vi "Create Read Write Stream.vi"(8 "error in (no error)":errorcluster, 10 "IP":string, 11 "Channel in":refnum<class "Channel.lvclass">) -> (0 "error out":errorcluster, 3 "Channel out":refnum<class "Channel.lvclass">)   [LabVIEW 2018, in "Channel.lvclass"]
uses:
  Channel.lvclass
  Stream/Stream.lvclass
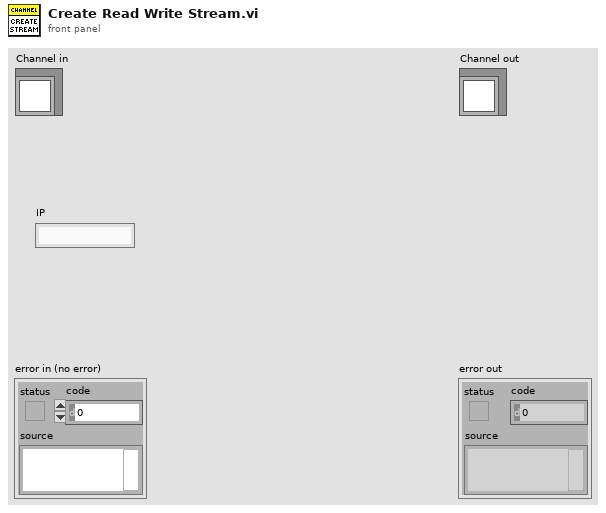
[diagram p1: front panel]
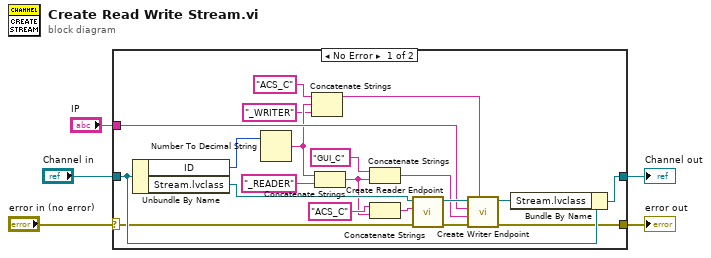
[diagram p0: block diagram]
diagram:
  n1 = case shown="No Error" "error in (no error)" {
    selector: "error in (no error)" -> [w23 w27]
    tunnel: [w20 w27] -> w4
    tunnel: [w24 w26] -> w2
    tunnel: "Channel in" -> [w25 w26]
    tunnel: "IP" -> [w17 _]
    frame No Error {
      n2 = Unbundle By Name(w25) -> ("ID"=w6:u8, "Stream.lvclass"=w22:refnum<class "Stream.lvclass">)
      n3 = Number To Decimal String(number=w6) -> (decimal integer string=w9:string)  [unwired: 1 in]
      n4 = Concatenate Strings("ACS_C" ("writer name"), w9, "_WRITER" ("writer name")) -> (w7:string)
      n5 = Concatenate Strings(w9, "_READER" ("writer name")) -> (w12:string)
      n6 = Concatenate Strings("GUI_C" ("writer name"), w12) -> (w11:string)
      n7 = Concatenate Strings("ACS_C" ("writer name"), w12) -> (w14:string)
      n8 = call "Create Reader Endpoint.vi"("error in (no error)"=w23, "reader name"=w14, "Stream in"=w22) -> ("error out"=w19:errorcluster, "Stream out"=w18:refnum<class "Stream.lvclass">)  [unwired: 7 in]
      n9 = call "Create Writer Endpoint.vi"(7:w7, "error in (no error)"=w19, "reader name"=w11, "IP"=w17, "Stream in"=w18) -> ("error out"=w20:errorcluster, "Stream out"=w21:refnum<class "Stream.lvclass">)  [unwired: 5 in]
      n10 = Bundle By Name(cluster=w25, "Stream.lvclass"=w21) -> (w24:refnum<class "Channel.lvclass">)
    }
    frame Error {
    }
  }
  "error out" <- w4
  "Channel out" <- w2
